vi "Read ourGoalPosition.vi"(8 "error in (no error)":errorcluster, 11 "Field in":refnum<class "Field.lvclass">) -> (0 "error out":errorcluster, 2 "ourGoalPosition":dbl[](array[numeric]), 3 "Field out":refnum<class "Field.lvclass">)   [LabVIEW 2021, in "Field.lvclass"]
uses:
  Field.lvclass
  Field.lvclass/Field.ctl
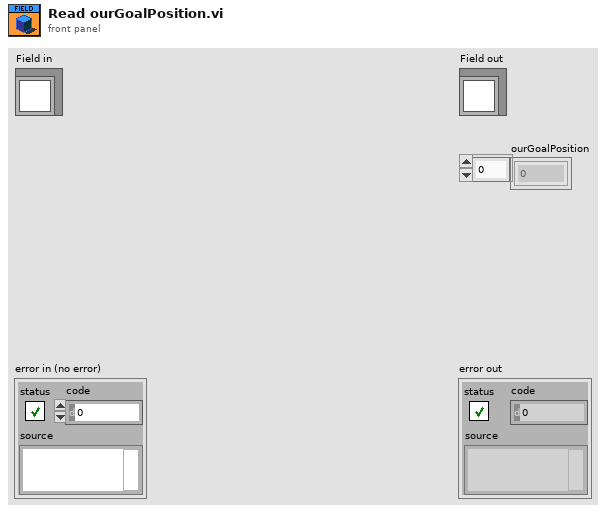
[diagram p1: front panel]
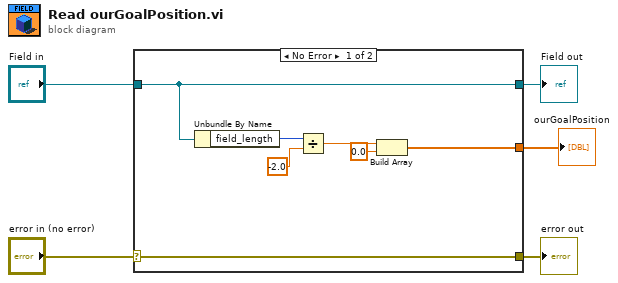
[diagram p0: block diagram]
diagram:
  n1 = case shown="No Error" "error in (no error)" {
    selector: "error in (no error)" -> [w12 w13]
    tunnel: [w12 w13] -> w4
    tunnel: [w7 w14] -> w2
    tunnel: "Field in" -> [w7 w14]
    tunnel: [w6 _] -> w1
    frame No Error {
      n2 = Unbundle By Name(w7) -> ("field_length"=w11:i32)
      n3 = Divide(x=w11, y=-2.0) -> (x/y=w9:dbl)
      n4 = Build Array(w9, 0.0 ("element")) -> (w6:dbl[])
    }
    frame Error {
    }
  }
  "error out" <- w4
  "Field out" <- w2
  "ourGoalPosition" <- w1
